vi "Draw.vi"(8 "error in (no error)":errorcluster, 11 "FSM in":refnum<class "FSM.Graph.lvclass">) -> (0 "error out":errorcluster, 2 "picture out":picture, 3 "FSM out":refnum<class "FSM.Graph.lvclass">)   [LabVIEW 2015, in "FSM.Graph.lvclass"]
uses:
  FSM.Graph.lvclass
  FSM.Graph.lvclass/FSM.Graph.ctl
  FSM.Node/FSM.Node.lvclass
  FSM.Edge/FSM.Edge.lvclass
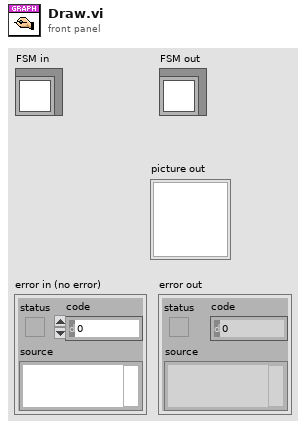
[diagram p1: front panel]
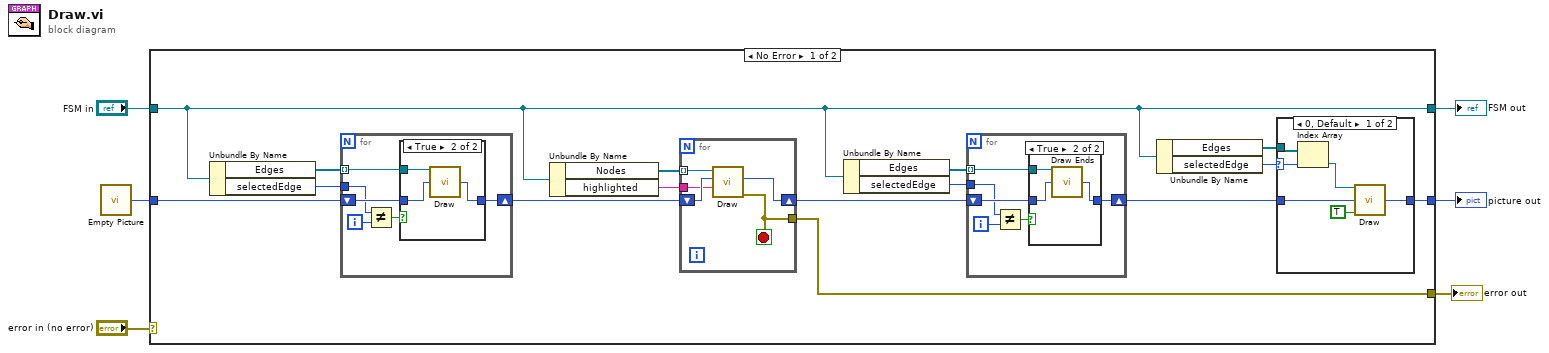
[diagram p0: block diagram]
diagram:
  n1 = call "Empty Picture"() -> ("empty picture"=w1:picture)
  n2 = case shown="No Error" "error in (no error)" {
    selector: "error in (no error)" -> [_ w56]
    tunnel: [w20 w56] -> w5
    tunnel: [w12 w55] -> w3
    tunnel: "FSM in" -> [w12 w55]
    tunnel: w1 -> [w18 w54]
    tunnel: [w10 w54] -> w2
    frame No Error {
      n3 = Unbundle By Name(w12) -> ("Edges"=w19:refnum<class "FSM.Edge.lvclass">[], "selectedEdge"=w14:i32)
      n4 = for {
        tunnel: w19 -> [w44] mode=indexing
        shift-right: [w42] -> w17
        shift-left: w18 -> [w43]
        tunnel: w14 -> [w40]
        i -> [w41]
        n5 = Not Equal?(x=w40, y=w41) -> (x != y?=w39:bool)
        n6 = case shown="True" w39 {
          tunnel: w44 -> [_ w48]
          tunnel: w43 -> [w45 w47]
          tunnel: [w45 w46] -> w42
          frame False {
          }
          frame True {
            n7 = call "Draw.vi"("FSM.Edge In"=w48, "picture in"=w47) -> ("picture out"=w46:picture)  [unwired: 12 in, 1 out]
          }
        }
      }
      n8 = Unbundle By Name(w12) -> ("Nodes"=w21:refnum<class "FSM.Node.lvclass">[], "highlighted"=w7:string)
      n9 = for {
        tunnel: w21 -> [w53] mode=indexing
        shift-right: [w51] -> w15
        shift-left: w17 -> [w52]
        tunnel: [w50] -> w20
        tunnel: w7 -> [w49]
        stop <- w50 stop-if-true
        n10 = call "Draw.vi"("Highlighted"=w49, "picture in"=w52, "FSM in"=w53) -> ("error out"=w50:errorcluster, "picture out"=w51:picture)  [unwired: 6 in, 1 out]
      }
      n11 = Unbundle By Name(w12) -> ("Edges"=w16:refnum<class "FSM.Edge.lvclass">[], "selectedEdge"=w13:i32)
      n12 = for {
        tunnel: w16 -> [w34] mode=indexing
        shift-right: [w32] -> w9
        shift-left: w15 -> [w33]
        tunnel: w13 -> [w30]
        i -> [w31]
        n13 = Not Equal?(x=w30, y=w31) -> (x != y?=w29:bool)
        n14 = case shown="True" w29 {
          tunnel: w34 -> [_ w38]
          tunnel: w33 -> [w35 w37]
          tunnel: [w35 w36] -> w32
          frame False {
          }
          frame True {
            n15 = call "Draw Ends.vi"("FSM.Edge In"=w38, "picture in"=w37) -> ("picture out"=w36:picture)  [unwired: 12 in, 1 out]
          }
        }
      }
      n16 = Unbundle By Name(w12) -> ("Edges"=w8:refnum<class "FSM.Edge.lvclass">[], "selectedEdge"=w11:i32)
      n17 = case shown="0, Default" w11 {
        selector: w11 -> [w27 _]
        tunnel: [w24 w28] -> w10
        tunnel: w9 -> [w25 w28]
        tunnel: w8 -> [w26 _]
        frame 0, Default {
          n18 = Index Array(array=w26, index=w27) -> (element=w23:refnum<class "FSM.Edge.lvclass">)
          n19 = call "Draw.vi"("FSM.Edge In"=w23, "picture in"=w25, "selected"=TRUE) -> ("picture out"=w24:picture)  [unwired: 11 in, 1 out]
        }
        frame -1 {
        }
      }
    }
    frame Error {
    }
  }
  "error out" <- w5
  "FSM out" <- w3
  "picture out" <- w2
